vi "timetest3.vi"() -> ()   [LabVIEW 2015]
uses:
  BERTTA.dll
panel:
  out "Waveform Chart":dynamicdata(graph)
  out "Current temp":dbl
  in  "Tset":dbl=50.0
  out "elapsed (float)":dbl
  out "elapsed (int)":i32
  out "setpoint":dbl
  in  "direction":i32
  out "element 6":i32
  in  "rt":i32=100
  out "element 5":i32
  out "element 4":i32
  out "element 3":i32
  out "element 2":i32
  out "element":i32
  in  "pause":i32
  in  "start":i32
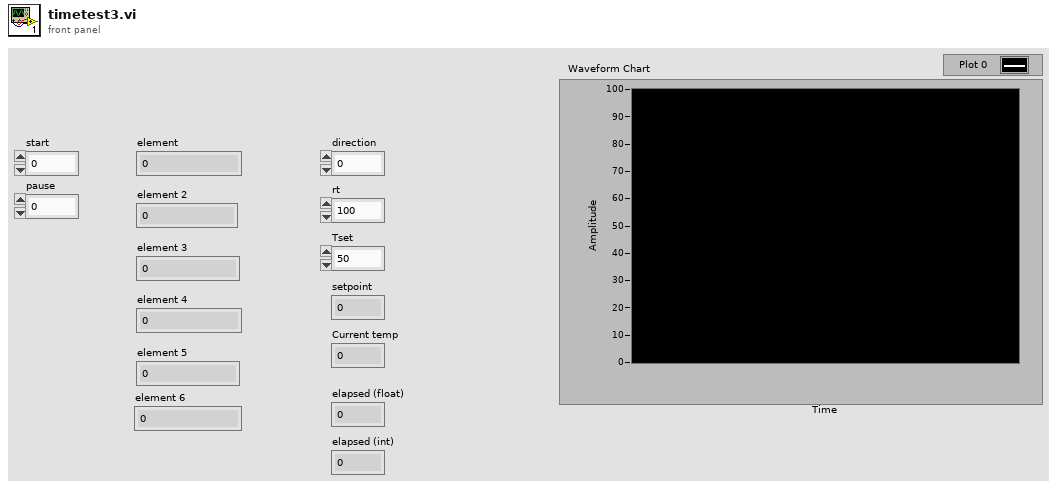
[diagram p1: front panel]
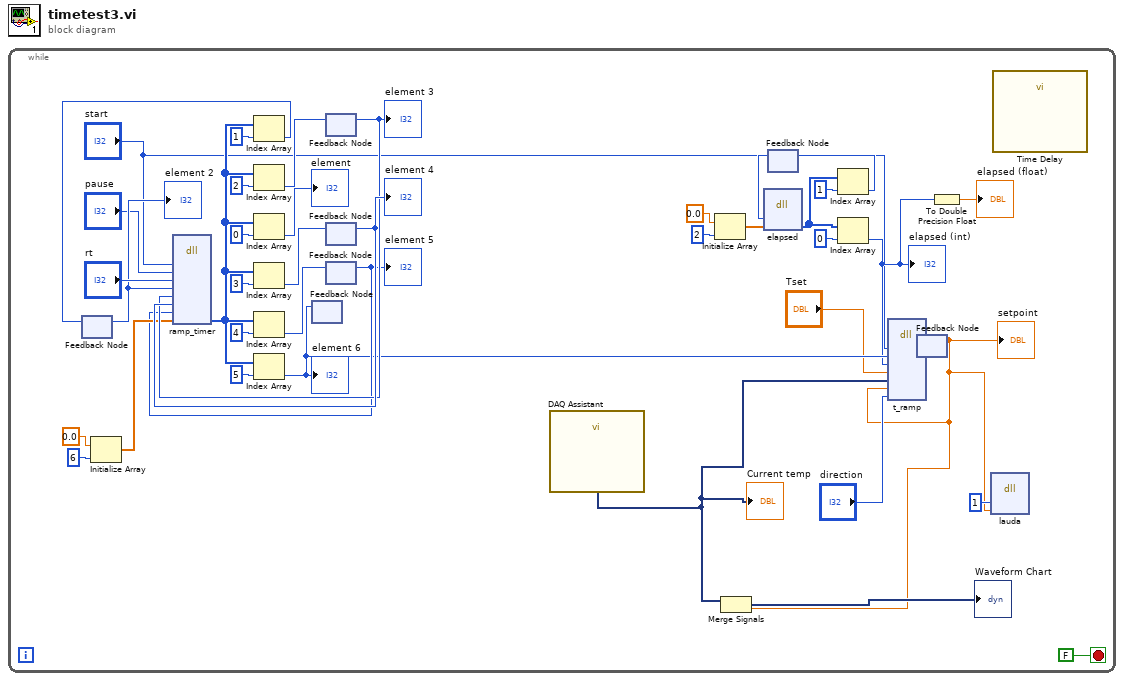
[diagram p0: block diagram]
diagram:
  n1 = while {
    stop <- FALSE stop-if-true
    n2 = feedback #1() -> (w31:i32)  [unwired: 1 in]
    "element 2" <- w31
    n3 = Initialize Array(0.0 ("element"), 6 ("dimension size")) -> (w23:dbl[])
    n4 = feedback #2() -> ()  [unwired: 2 in]
    n5 = feedback #3() -> (w33:i32)  [unwired: 1 in]
    "element 3" <- w33
    n6 = feedback #4() -> (w36:i32)  [unwired: 1 in]
    "element 4" <- w36
    n7 = feedback #5() -> (w21:i32)  [unwired: 1 in]
    "element 5" <- w21
    n8 = dll-call lib="C:/Users/xlaraser/Documents/Visual Studio 2017/Projects/Bertta/BERTTA/Debug/BERTTA.dll" fn="ramp_timer"("enable"="start", "pause"="pause", "rt"="rt", "start_time"=w31, "pause_time"=w33, "paused"=w36, "paused_old"=w21, "params"=w23) -> ("params"=w41:i32[])  [unwired: 11 in, 2 out]
    n9 = Index Array(array=w41, index=1) -> (element=w30:i32)
    n10 = feedback-in #1(w30) -> ()
    n11 = Index Array(array=w41, index=2) -> (element=w32:i32)
    n12 = Index Array(array=w41, index=0) -> (element=→"element":i32)
    n13 = Index Array(array=w41, index=3) -> (element=w35:i32)
    n14 = Index Array(array=w41, index=4) -> (element=w38:i32)
    n15 = Index Array(array=w41, index=5) -> (element=w11:i32)
    "element 6" <- w11
    n16 = feedback-in #2(w11) -> ()
    n17 = feedback-in #3(w32) -> ()
    n18 = feedback-in #4(w35) -> ()
    n19 = feedback-in #5(w38) -> ()
    n20 = call "DAQ Assistant"() -> ("data"=w4:dynamicdata)  [unwired: 17 in, 2 out]
    "Current temp" <- w4
    n21 = Initialize Array(0.0 ("element"), 2 ("dimension size")) -> (w19:dbl[])
    n22 = feedback #6() -> (w12:i32)  [unwired: 1 in]
    n23 = dll-call lib="C:/Users/xlaraser/Documents/Visual Studio 2017/Projects/Bertta/BERTTA/Debug/BERTTA.dll" fn="elapsed"("last_time"=w12, "params"=w19) -> ("params"=w15:i32[])  [unwired: 5 in, 2 out]
    n24 = Index Array(array=w15, index=1) -> (element=w13:i32)
    n25 = feedback-in #6(w13) -> ()
    n26 = Index Array(array=w15, index=0) -> (element=w9:i32)
    "elapsed (int)" <- w9
    n27 = feedback #7() -> (w2:dbl)  [unwired: 1 in]
    "setpoint" <- w2
    n28 = Merge Signals(w4, w2) -> (→"Waveform Chart":dynamicdata)
    n29 = dll-call lib="C:/Users/xlaraser/Documents/Visual Studio 2017/Projects/Bertta/BERTTA/Debug/BERTTA.dll" fn="t_ramp"("enable"="start", "ramp_time"=w11, "elapsed"=w9, "Tset"="Tset", "Tcurrent"=w4, "Tcurr_prev"=w2, "direction"="direction") -> ("return type"=w5:dbl)  [unwired: 10 in, 2 out]
    n30 = feedback-in #7(w5) -> ()
    n31 = To Double Precision Float(number=w9) -> (double precision float=→"elapsed (float)":dbl)
    n32 = dll-call lib="C:/Users/xlaraser/Documents/Visual Studio 2017/Projects/Bertta/BERTTA/Debug/BERTTA.dll" fn="lauda"("port"=1, "set_temp"=w2) -> ()  [unwired: 6 in, 2 out]
    n33 = call "Time Delay"() -> ()  [unwired: 11 in, 1 out]
  }
